vi "Get Value of LabVIEW Cluster.vi"(8 "error in (no error)":errorcluster, 10 "LabVIEW Cluster":refnum<vi>) -> (0 "error out":errorcluster, 3 "JSON Tree Object Out":variant)   [LabVIEW 2011, in "i3-json.lvlib"]
doc: "This VI takes a JSON Node (all types besides JSON Object) and assigns the value to the LabVIEW Base Type of compatible reference.\n\nIf the LabVIEW base type is an array of boolean, numeric, or string this function will attempt to check if a JSON Array type will map"
uses:
  i3-json.lvlib
  JSON Types/JSON Type.ctl
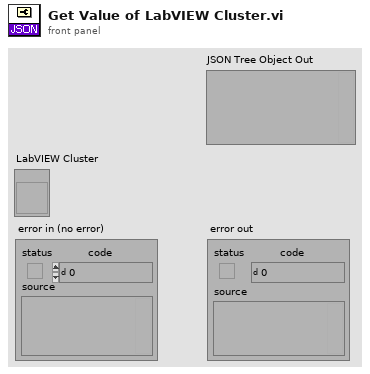
[diagram p1: front panel]
types:
  T1 = typedef "i3-json.lvlib/JSON Type.ctl" = enum8{"JSON Compatible", "JSON Array", "JSON Object", "JSON Null", "Double", "String", "Boolean", "Unknown", "Data JSON string"}
  T2 = typedef "Type Enum.ctl" = enum8{"Void", "I8", "I16", "I32", "I64", "U8", "U16", "U32", "U64", "Single Float", "Double Float", "Extended Float", "Single Complex", "Double Complex", "Extended Complex", "Enum I8 NEVER", "Enum I16 NEVER", "Enum I32 NEVER", "Enum I64 NEVER", "Enum U8", "Enum U16", "Enum U32", "Enum U64", "Single Float With Unit", "Double Float With Unit", "Extended Float With Unit", "Single Complex With Unit", "Double Complex With Unit", "Extended Complex With Unit", "boolU16", "Boolean", "String", "Handle", "Path", "Picture", "C String", "Pascal String", "Tag", "SubString", "Array", "SubArray", "Cluster", "Numeric Cluster", "Variant", "LV Variant", "Measure Data (waveform)", "Refnum", "ExtData", "function", "Typedef", "Poly VI", "bad wire", "LabVIEW Class Instance"}
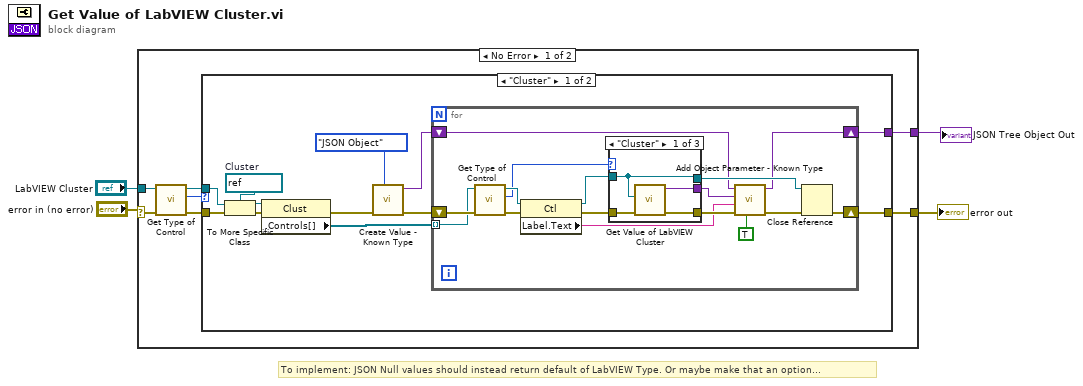
[diagram p0: block diagram]
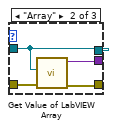
[diagram p2: hidden frame]
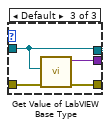
[diagram p3: hidden frame]
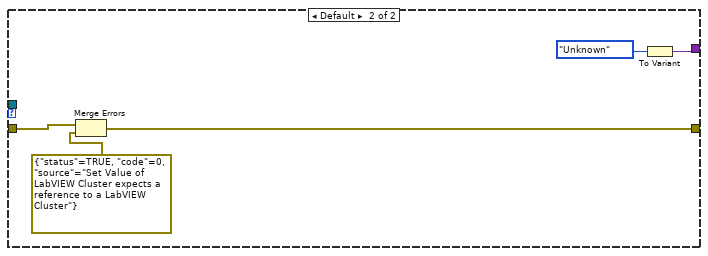
[diagram p4: hidden frame]
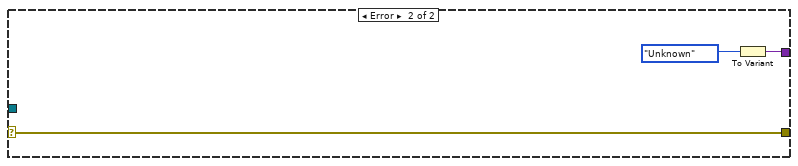
[diagram p5: hidden frame]
diagram:
  # "To implement: JSON Null values should instead return default of LabVIEW Type. Or maybe make that an option..."
  n1 = case shown="No Error" "error in (no error)" {
    selector: "error in (no error)" -> [w11 w59]
    tunnel: "LabVIEW Cluster" -> [w10 _]
    tunnel: [w6 w59] -> w2
    tunnel: [w5 w58] -> w1
    frame No Error {
      n2 = call <vilib>:"Get Type of Control.vi"("error in (no error)"=w11, "Control Ref In"=w10) -> ("error out"=w7:errorcluster, "Type Enum"=w9:T2, "Control Ref Out"=w8:refnum<vi>)  [unwired: 7 in]
      n3 = case shown="\"Cluster\"" w9 {
        tunnel: w8 -> [w22 _]
        tunnel: w7 -> [w23 w56]
        tunnel: [w17 w54] -> w6
        tunnel: [w12 w53] -> w5
        frame "Cluster" {
          w20 = refnum<vi> refnum  # Cluster
          n4 = To More Specific Class(target class=w20, reference=w22, error in=w23) -> (specific class reference=w19:refnum<vi>, error out=w21:errorcluster)
          n5 = property class="Clust"(reference=w19, error in=w21) -> (error out=w16:errorcluster, "Controls[]"=w18:refnum<vi>[])  [unwired: 1 out]
          n6 = call "Create Value - Known Type.vi"("JSON Type"=JSON_Type."JSON Object", "error in (no error)"=w16) -> ("error out"=w15:errorcluster, "JSON Tree"=w13:variant)  [unwired: 8 in]
          n7 = for {
            tunnel: w18 -> [w38] mode=indexing
            shift-right: [w33] -> w17
            shift-left: w15 -> [w39]
            shift-right: [w24] -> w12
            shift-left: w13 -> [w26]
            n8 = call <vilib>:"Get Type of Control.vi"("error in (no error)"=w39, "Control Ref In"=w38) -> ("error out"=w36:errorcluster, "Type Enum"=w34:T2, "Control Ref Out"=w37:refnum<vi>)  [unwired: 7 in]
            n9 = property class="Ctl"(reference=w37, error in=w36) -> (reference out=w35:refnum<vi>, error out=w31:errorcluster, "Label.Text"=w27:string)
            n10 = case shown="\"Cluster\"" w34 {
              tunnel: [w43 w47 w51] -> w30
              tunnel: w35 -> [w42 w46 w50]
              tunnel: [w42 w46 w50] -> w32
              tunnel: w31 -> [w41 w45 w49]
              tunnel: [w40 w44 w48] -> w28
              frame "Cluster" {
                n11 = call "Get Value of LabVIEW Cluster.vi"("error in (no error)"=w41, "LabVIEW Cluster"=w42) -> ("error out"=w43:errorcluster, "JSON Tree Object Out"=w40:variant)  [unwired: 8 in]
              }
              frame "Array" {
                n12 = call "Get Value of LabVIEW Array.vi"("LabVIEW Array"=w46, "error in (no error)"=w45) -> ("JSON Tree Array"=w44:variant, "error out"=w47:errorcluster)  [unwired: 7 in]
              }
              frame Default {
                n13 = call "Get Value of LabVIEW Base Type.vi"("LabVIEW Base Type"=w50, "error in (no error)"=w49) -> ("JSON Tree Out"=w48:variant, "error out"=w51:errorcluster)  [unwired: 7 in]
              }
            }
            n14 = call "Add Object Parameter - Known Type.vi"("Add Parameter as JSON Tree?"=TRUE, "error in (no error)"=w30, "Name"=w27, "Value"=w28, "JSON Tree in (JSON Object)"=w26) -> ("error out"=w29:errorcluster, "JSON Tree out (JSON Object)"=w24:variant)  [unwired: 5 in]
            n15 = Close Reference(reference=w32, error in (no error)=w29) -> (error out=w33:errorcluster)
          }
        }
        frame Default {
          n16 = Merge Errors(w56, errorcluster {"status"=TRUE, "code"=0, "source"="Set Value of LabVIEW Cluster expects a reference to a LabVIEW Cluster"} ("error in")) -> (w54:errorcluster)
          n17 = To Variant(anything=JSON_Type."Unknown" ("JSON Type")) -> (Variant=w53:variant)
        }
      }
    }
    frame Error {
      n18 = To Variant(anything=JSON_Type."Unknown" ("JSON Type")) -> (Variant=w58:variant)
    }
  }
  "JSON Tree Object Out" <- w1
  "error out" <- w2
